vi "Untitled 1.vi"() -> ()   [LabVIEW 2017]
uses:
  44f9835a-746c-4539-bace-5809b1497f9b.vi
  addons/API-String-Arugments-Support/API String Arguments Support.lvlib
panel:
  out "Cluster":cluster{"2d":dbl[][]}={"2d"=[[3.12, 4.113, 2.3, 5.0, 5.0, 2.3, 4.11, 5.0]]}
  out "error 13":errorcluster
  in  "String 13":string="[3.12,4.113,2.3,5;3.12,5,2.3;3.12,4.11,5]"
  out "Data 6":enum16{"1 - aaaa", "2 - bbbb", "555 - ccccc"}(ring)=enum."555 - ccccc"
  out "error 6":errorcluster
  in  "String 6":string="555"
  out "String":string
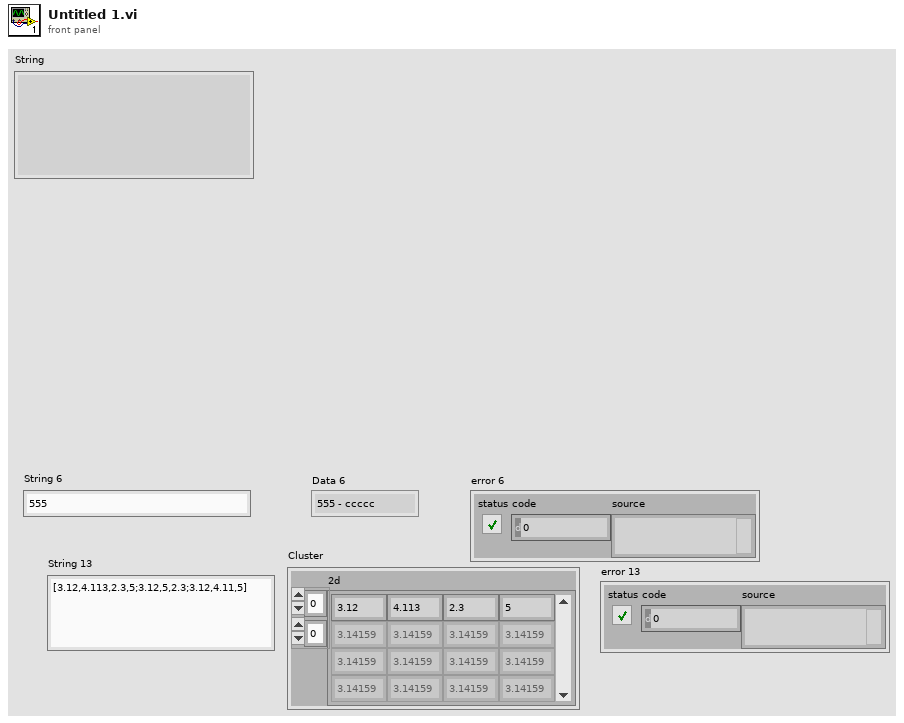
[diagram p1: front panel]
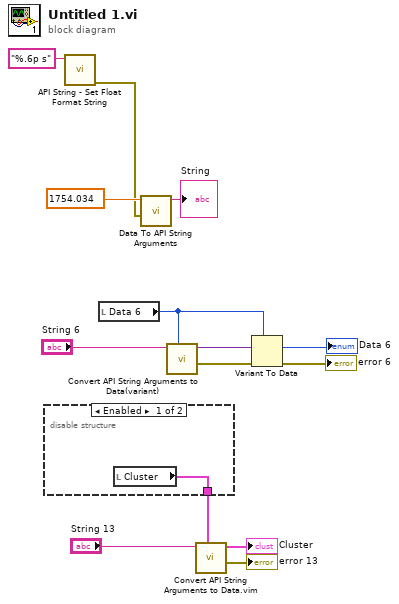
[diagram p0: block diagram]
diagram:
  n1 = disable-structure shown="Enabled" {
    disable-tunnel: [w15 _] -> w4
    frame Enabled {
      n2 = local read "Cluster"() -> (w15:cluster{"2d":dbl[][]})
    }
    frame Disabled {
    }
  }
  n3 = call "API String - Set Float Format String.vi"("Float Format String Setting"="%.6p s") -> ("Error out"=w1:errorcluster)  [unwired: 9 in, 1 out]
  n4 = local read "Data 6"() -> (w12:enum16{"1 - aaaa", "2 - bbbb", "555 - ccccc"})
  n5 = call "Data To API String Arguments.vi"("error in (no error)"=w1, "data"=1754.034) -> ("String"=→"String":string)  [unwired: 8 in, 1 out]
  n6 = call "Convert API String Arguments to Data(variant).vi"("Type"=w12, "String"="String 6") -> ("error"=w8:errorcluster, "Data"=w9:variant)  [unwired: 8 in]
  n7 = call "Convert API String Arguments to Data.vim"("Reference Type"=w4, "API String"="String 13") -> ("error out"=→"error 13":errorcluster, "Data"=→"Cluster":cluster{"2d":dbl[][]})  [unwired: 6 in]
  n8 = Variant To Data(error in=w8, type=w12, Variant=w9) -> (data=→"Data 6":enum16{"1 - aaaa", "2 - bbbb", "555 - ccccc"}, error out=→"error 6":errorcluster)
